vi "readImage.vi"(8 "Error in":errorcluster, 9 "raster":u8[](array[numeric]), 10 "tif":i64, 11 "Image Number":i32) -> (0 "Error Out":errorcluster, 1 "error":i32, 2 "tif pointer":i64, 3 "pixels":u8[](array[numeric]))   [LabVIEW 2013]
uses:
  imagereconstruction/x64/Debug/labviewdll.dll
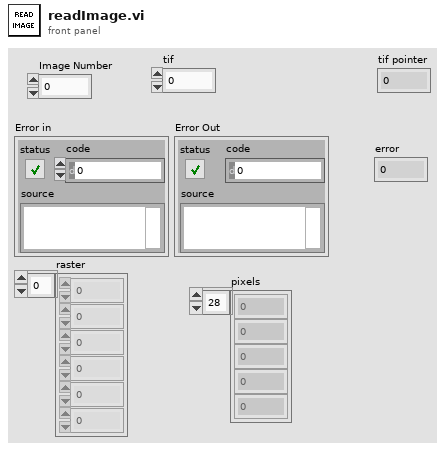
[diagram p1: front panel]
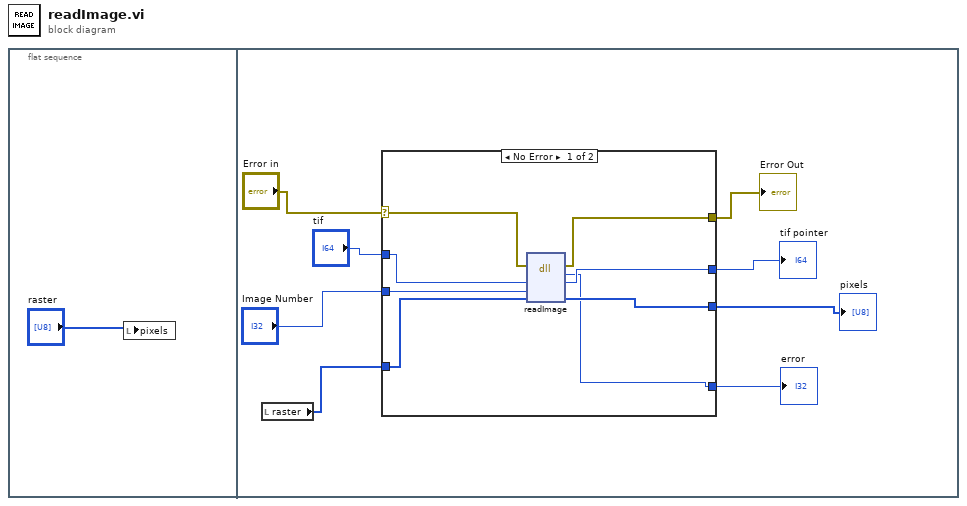
[diagram p0: block diagram]
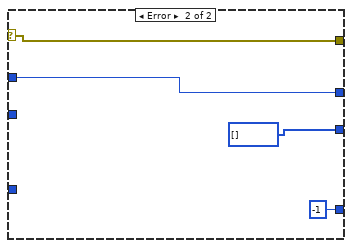
[diagram p2: hidden frame]
diagram:
  n1 = flat-sequence {
    frame #0 {
      n2 = local write "pixels"("raster") -> ()
    }
    frame #1 {
      n3 = local read "raster"() -> (w2:u8[])
      n4 = case shown="No Error" "Error in" {
        selector: "Error in" -> [w16 w21]
        tunnel: [w15 w21] -> w8
        tunnel: "Image Number" -> [w17 _]
        tunnel: w2 -> [w12 _]
        tunnel: "tif" -> [w13 w20]
        tunnel: [w14 w20] -> w5
        tunnel: [w10 -1 ("error")] -> w4
        tunnel: [w11 u8[] [] ("raster")] -> w3
        frame No Error {
          n5 = dll-call lib="D:/work/uni/FYP/reconrepo/imagereconstruction/x64/Debug/labviewdll.dll" fn="readImage"(error in=w16, "tif"=w13, "directory"=w17, "pixels"=w12) -> (error out=w15:errorcluster, "return type"=w10:i32, "tif"=w14:i64, "pixels"=w11:u8[])  [unwired: 3 in, 1 out]
        }
        frame Error {
        }
      }
      "Error Out" <- w8
      "pixels" <- w3
      "tif pointer" <- w5
      "error" <- w4
    }
  }
